vi "Update Start Button State.vi"(8 "error in (no error)":errorcluster, 10 "Start Button State":bool, 11 "Simulated Entry Console in":refnum<class "Simulated Entry Console.lvclass">) -> (0 "error out":errorcluster, 3 "Simulated Entry Console out":refnum<class "Simulated Entry Console.lvclass">)   [LabVIEW 2012, in "Simulated Entry Console.lvlib" / "Simulated Entry Console.lvclass"]
uses:
  Simulated Entry Console.lvclass
  Entry Console API/Entry Console API/Entry Console API.lvclass
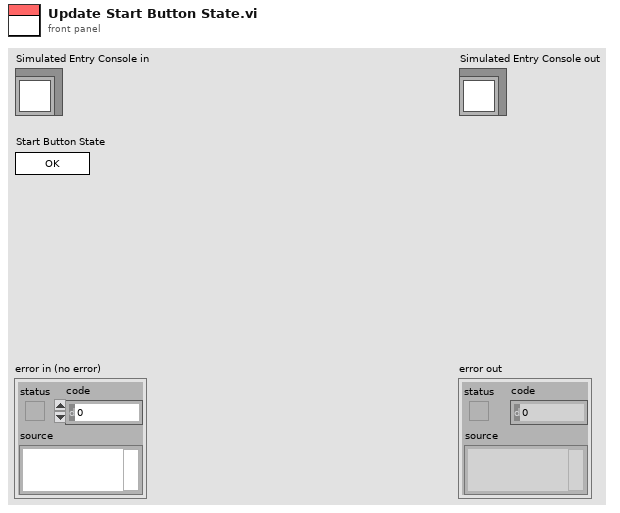
[diagram p1: front panel]
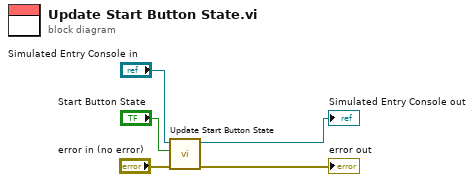
[diagram p0: block diagram]
diagram:
  n1 = call-parent "Update Start Button State.vi"("error in (no error)"="error in (no error)", "Start Button State"="Start Button State", "Entry Console API in"="Simulated Entry Console in") -> ("error out"=→"error out":errorcluster, "Entry Console API out"=→"Simulated Entry Console out":refnum<class "Simulated Entry Console.lvclass">)  [unwired: 7 in]
